vi "Read Measurement Osciloscope.vi"(8 "error in (no error)":errorcluster, 10 "Read Measurement In":T1={"TEKTRONIX- READ-IN"={"Channel (1: Channel 1)"=1, "Measurement Type (0: Frequency)"=0}, "EDU-X-1200A- READ-IN"={"Slope Type (0: Positive)"=0, "Measurement Type (0: Peak-Peak)"=0, "Occurrence Value (1)"=1, "Vertical Cross Value (0)"=0.0}} {"EDU-X-1200A- READ-IN"."Measurement Type (0: Peak-Peak)" items=["Peak-Peak", "Maximum", "Minimum", "Amplitude", "Top", "Base", "Overshoot", "Preshoot", "Average - N Cycles", "Average - Full Screen", "DC RMS - N Cycles", "DC RMS - Full Screen", "AC RMS - N Cycles", "AC RMS - Full Screen (Std Dev)", "Ratio", "Period", "Frequency", "Counter", "+Width", "-Width", "Burst Width", "Duty Cycle", "Rise Time", "Fall Time", "Delay", "Phase", "X minY", "X maxY", "Positive Pulse Count", "Negative Pulse Count", "Raising Edge Count", "Falling Edge Count", "Area - N Cycle", "Area - Full Screen", "Nth Edge Time", "Nth Edge Cross Level Time"]; "EDU-X-1200A- READ-IN"."Slope Type (0: Positive)" items=["Positive", "Negative"]; "TEKTRONIX- READ-IN"."Measurement Type (0: Frequency)" items=["Frequency", "Mean", "Period", "Pulse Duty", "Peak to Peak", "Cycle RMS", "Minimum", "Maximum", "Rise Time", "Fall Time", "Positive Width", "Negative Width", "Amplitude", "Cycle Mean", "High", "Low", "Negative Duty", "Positive Overshoot", "Negative Overshoot", "Cursor Mean", "Burst Width", "Positive Pulse Count", "Negative Pulse Count", "Rising Edge Count", "Falling Edge Count", "Area", "Cycle Area", "RMS", "Cursor RMS"]; "TEKTRONIX- READ-IN"."Channel (1: Channel 1)" items=["Channel 1"=1, "Channel 2"=2, "Channel 3"=3, "Channel 4"=4]}, 11 "OsciloscopeClass in":refnum<class "OsciloscopeClass.lvclass">) -> (0 "error out":errorcluster, 2 "Read measurement Out":T2, 3 "OsciloscopeClass out":refnum<class "OsciloscopeClass.lvclass">)   [LabVIEW 2020, in "OsciloscopeClass.lvclass"]
uses:
  OsciloscopeClass.lvclass
  TypeDefs/ReadMeasurementOut--cluster.ctl
  TypeDefs/ReadMeasurementIn--cluster.ctl
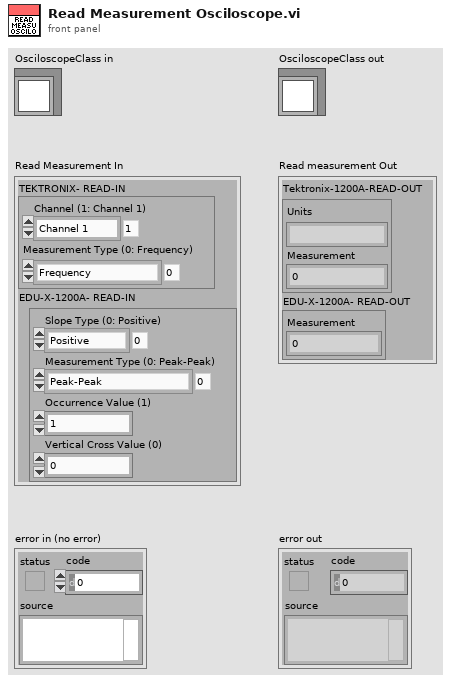
[diagram p1: front panel]
types:
  T1 = typedef "ReadMeasurementIn--cluster.ctl" = cluster{"TEKTRONIX- READ-IN":cluster{"Channel (1: Channel 1)":i32, "Measurement Type (0: Frequency)":i32}, "EDU-X-1200A- READ-IN":cluster{"Slope Type (0: Positive)":i32, "Measurement Type (0: Peak-Peak)":i32, "Occurrence Value (1)":i32, "Vertical Cross Value (0)":dbl}}
  T2 = typedef "ReadMeasurementOut--cluster.ctl" = cluster{"Tektronix-1200A-READ-OUT":cluster{"Units":string, "Measurement":dbl}, "EDU-X-1200A- READ-OUT":cluster{"Measurement":dbl}}
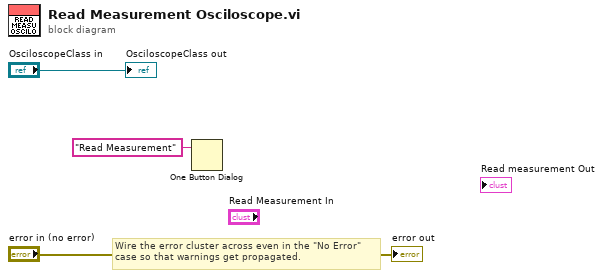
[diagram p0: block diagram]
diagram:
  # "Wire the error cluster across even in the \"No Error\"\ncase so that warnings get propagated."
  n1 = One Button Dialog(message="Read Measurement") -> ()  [unwired: 1 in, 1 out]
  "error out" <- "error in (no error)"
  "OsciloscopeClass out" <- "OsciloscopeClass in"
